vi "Acquire.vi"(4 "Acquisition Status Notifier":refnum<notifier>, 6 "Force?":bool, 8 "error in (no error)":errorcluster, 9 "Data Queue":refnum<queue>, 10 "Data Notifier":refnum<notifier>, 11 "Hardware Resources in":T1) -> (0 "error out":errorcluster, 3 "Hardware Resources out":T1)   [LabVIEW 2021, in "Acquisition.lvlib"]
doc: "Perform the acquisition. Replace the contents of this diagram with calls to acquisition hardware."
uses:
  Acquisition.lvlib
  Hardware Configuration.ctl
  Channel Settings.ctl
  IO Device.ctl
  Interval Timer/Repeat Interval.ctl
  Interval Timer/Interval Length.ctl
  Interval Timer/Interval Token.ctl
  controls/Acquired Data.ctl
  controls/Acquisition Status.ctl
  Interval Timer/Interval Timer.lvlib
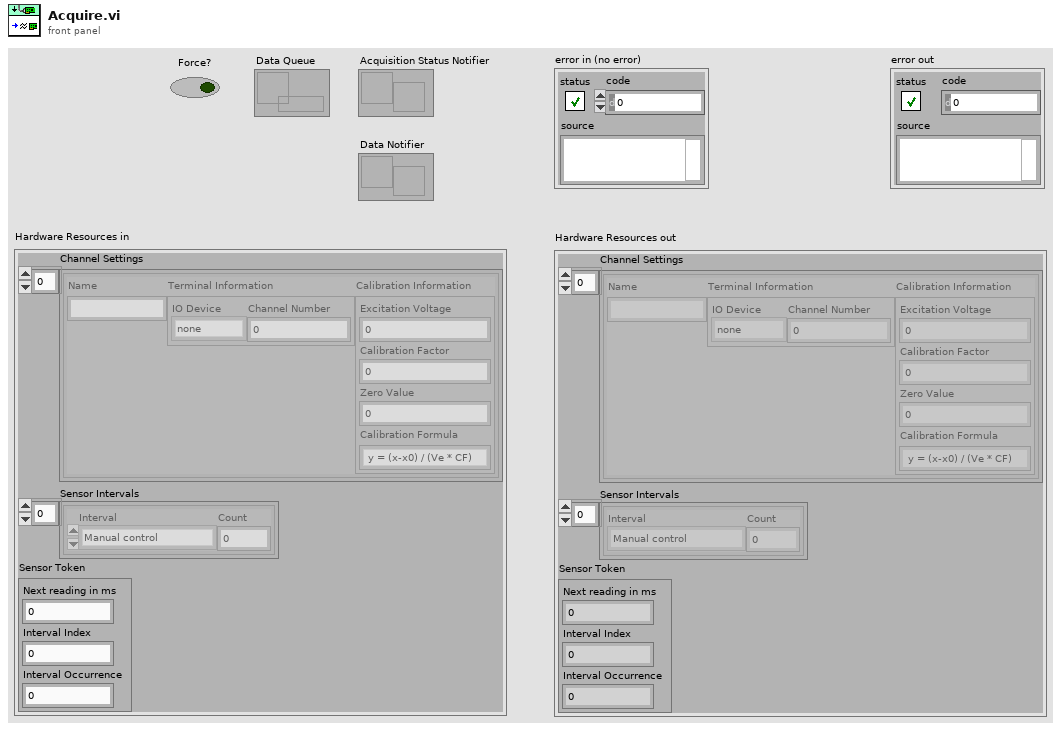
[diagram p1: front panel]
types:
  T1 = typedef "Acquisition.lvlib/Hardware Configuration.ctl" = cluster{"Channel Settings":T2[], "Sensor Intervals":T4[], "Sensor Token":T6}
  T2 = typedef "Acquisition.lvlib/Channel Settings.ctl" = cluster{"Name":string, "Terminal Information":cluster{"IO Device":T3, "Channel Number":i32}, "Calibration Information":cluster{"Excitation Voltage":dbl, "Calibration Factor":dbl, "Zero Value":dbl, "Calibration Formula":string}}
  T3 = typedef "Acquisition.lvlib/IO Device.ctl" = enum16{"none", "9219", "9401"}
  T4 = typedef "Interval Timer.lvlib/Repeat Interval.ctl" = cluster{"Interval":T5, "Count":i32}
  T5 = typedef "Interval Timer.lvlib/Interval Length.ctl" = enum16{"Manual control", "1 second", "10 seconds", "30 seconds", "60 seconds", "600 seconds", "1200 seconds", "3600 seconds"}
  T6 = typedef "Interval Timer.lvlib/Interval Token.ctl" = cluster{"Next reading in ms":u32, "Interval Index":i32, "Interval Occurrence":i32}
  T7 = typedef "Acquired Data.ctl" = cluster{"Waveform Array":waveform(dbl)[]}
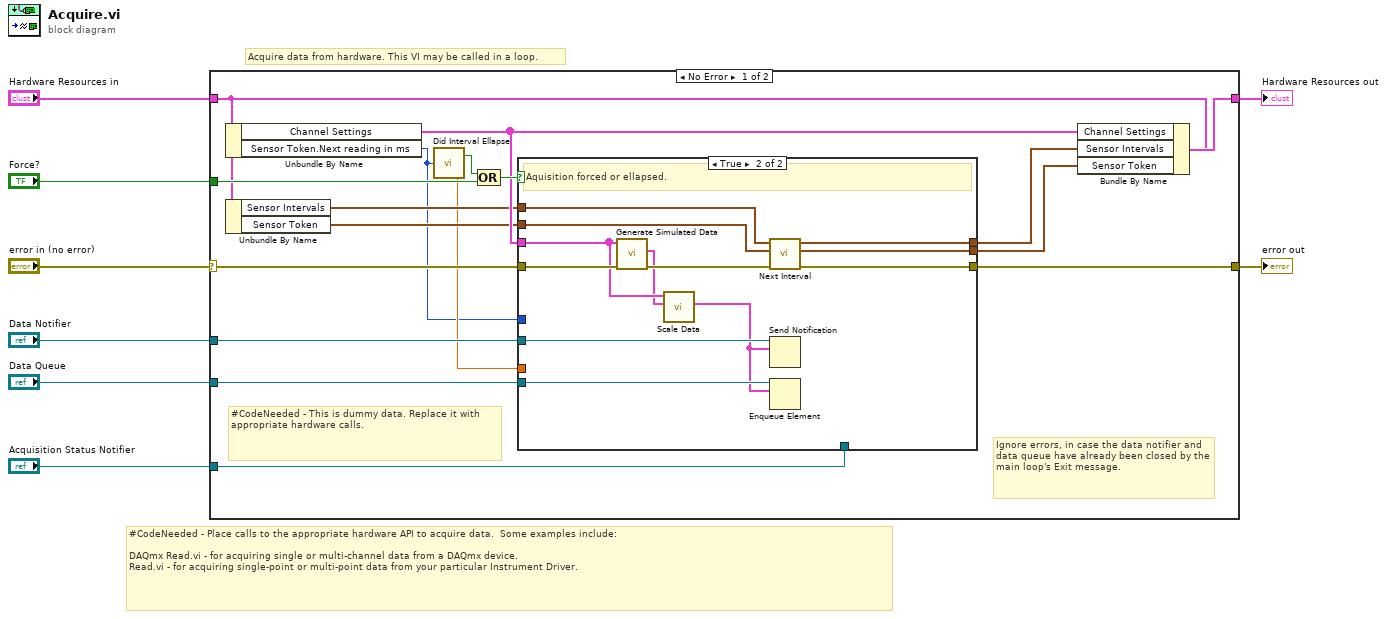
[diagram p0: block diagram]
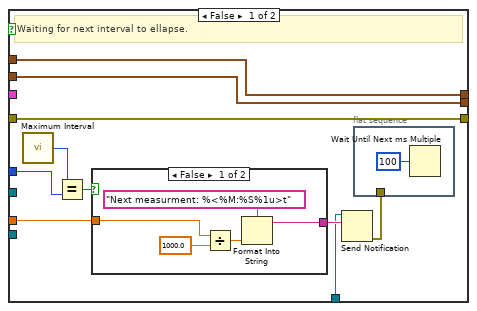
[diagram p2: hidden frame]
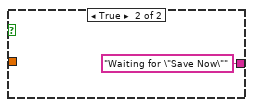
[diagram p3: hidden frame]
diagram:
  # "Acquire data from hardware. This VI may be called in a loop."
  # "#CodeNeeded - Place calls to the appropriate hardware API to acquire data.  Some examples include:\n\nDAQmx Read.vi - for acquiring single or multi-channel data from a DAQmx device.\nRead.vi - for acquiring single-point or multi-point data from your particular Instrument Driver."
  n1 = case shown="No Error" "error in (no error)" {
    selector: "error in (no error)" -> [w21 w55]
    tunnel: [w19 w55] -> w7
    tunnel: "Hardware Resources in" -> [w16 w56]
    tunnel: [w25 w56] -> w5
    tunnel: "Data Notifier" -> [w17 _]
    tunnel: "Data Queue" -> [w18 _]
    tunnel: "Force?" -> [w23 _]
    tunnel: "Acquisition Status Notifier" -> [w11 _]
    frame No Error {
      # "Ignore errors, in case the data notifier and data queue have already been closed by the main loop's Exit message."
      # "#CodeNeeded - This is dummy data. Replace it with appropriate hardware calls."
      n2 = Unbundle By Name(w16) -> ("Channel Settings"=w20:T2[], "Sensor Token.Next reading in ms"=w9:u32)
      n3 = Unbundle By Name(w16) -> ("Sensor Intervals"=w15:T4[], "Sensor Token"=w14:T6)
      n4 = call "Did Interval Ellapse.vi"("Future time coordinate (ms)"=w9) -> ("ms Until Next"=w10:dbl, "Interval Ellapsed?"=w24:bool)  [unwired: 2 in]
      n5 = Compound Arithmetic op=OR(w24, w23) -> (w22:bool)
      n6 = case shown="True" w22 {
        tunnel: w21 -> [w35 w54]
        tunnel: w20 -> [_ w45]
        tunnel: [w35 w50] -> w19
        tunnel: w18 -> [_ w53]
        tunnel: w17 -> [_ w52]
        tunnel: w15 -> [w34 w49]
        tunnel: w14 -> [w33 w48]
        tunnel: [w34 w47] -> w13
        tunnel: [w33 w46] -> w12
        tunnel: w11 -> [w30 _]
        tunnel: w10 -> [w29 _]
        tunnel: w9 -> [w26 _]
        frame False {
          # "Waiting for next interval to ellapse."
          n7 = call "Maximum Interval.vi"() -> ("New Acquisition Time"=w28:u32)
          n8 = Equal?(x=w28, y=w26) -> (x = y?=w27:bool)
          n9 = case shown="False" w27 {
            tunnel: [w39 "Waiting for \"Save Now\""] -> w32
            tunnel: w29 -> [w38 _]
            frame False {
              n10 = Divide(x=w38, y=1000.0) -> (x/y=w37:dbl)
              n11 = Format Into String(format string="Next measurment: %<%M:%S%1u>t", w37) -> (resulting string=w39:string)  [unwired: 2 in, 1 out]
            }
            frame True {
            }
          }
          n12 = Send Notification(notification=w32, notifier=w30) -> (error out=w31:errorcluster)  [unwired: 1 in, 1 out]
          n13 = flat-sequence {
            tunnel: w31 -> [_]
            frame #0 {
              n14 = Wait Until Next ms Multiple(millisecond multiple=u32 100) -> ()  [unwired: 1 out]
            }
          }
        }
        frame True {
          # "Aquisition forced or ellapsed."
          n15 = call "Generate Simulated Data.vi"("error in (no error)"=w54, "Channel Settings"=w45) -> ("error out"=w51:errorcluster, "Graph Data"=w44:T7)  [unwired: 8 in]
          n16 = call "Scale Data.vi"("Raw Graph Data"=w44, "Channel Settings"=w45) -> ("Scaled Graph Data"=w43:T7)  [unwired: 9 in]
          n17 = call "Next Interval.vi"("error in"=w51, "Interval Token in"=w48, "Intervals in"=w49) -> ("error out"=w50:errorcluster, "Interval Token out"=w46:T6, "Intervals out"=w47:T4[])  [unwired: 5 in, 1 out]
          n18 = Send Notification(notification=w43, notifier=w52) -> ()  [unwired: 1 in, 2 out]
          n19 = Enqueue Element(queue=w53, element=w43) -> ()  [unwired: 2 in, 3 out]
        }
      }
      n20 = Bundle By Name(cluster=w16, "Channel Settings"=w20, "Sensor Intervals"=w13, "Sensor Token"=w12) -> (w25:T1)
    }
    frame Error {
    }
  }
  "Hardware Resources out" <- w5
  "error out" <- w7
